vi "calculate_white-bias_jsc.vi"(9 "wavelengths":dbl[](array[numeric]), 10 "eqe measurements":dbl[](array[numeric]), 11 "am1.5 jsc (mA/cm^2)":dbl) -> (2 "white bias (# of suns)":dbl)   [LabVIEW 2018]
uses:
  <vilib>/Analysis/2dsp.llb/Integral Method.ctl
  <vilib>/Analysis/8numeric.llb/1D Numeric Integration.vi
  <vilib>/Utility/file.llb/Read Delimited Spreadsheet (DBL).vi
  <vilib>/gmath/NI_Gmath.lvlib
  <vilib>/Analysis/NI_AALPro.lvlib
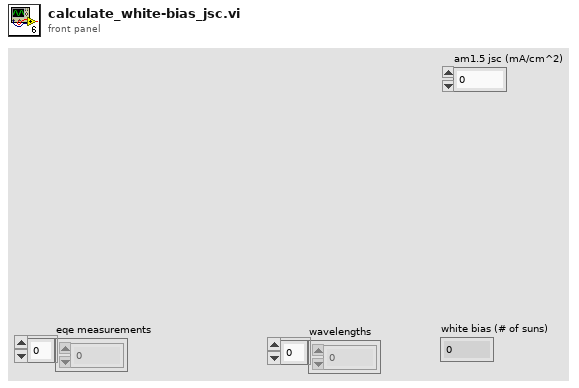
[diagram p1: front panel]
types:
  T1 = typedef "NI_AALPro.lvlib/Integral Method.ctl" = i32
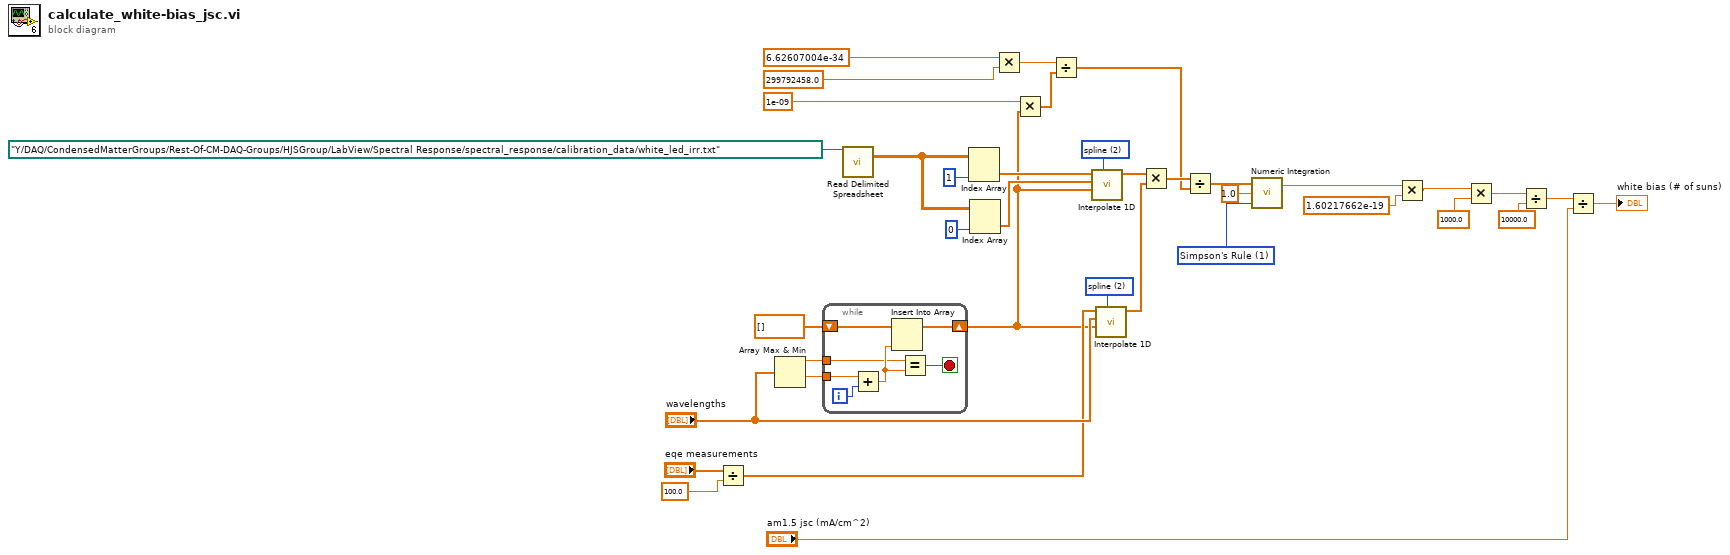
[diagram p0: block diagram]
diagram:
  w10 = 2 items=["nearest", "linear", "spline", "cubic Hermite", "Lagrange"] ("method")
  w18 = T1 1 items=["Trapezoidal Rule", "Simpson's Rule", "Simpson's 3/8 Rule", "Bode Rule"] ("integration method")
  w31 = 2 items=["nearest", "linear", "spline", "cubic Hermite", "Lagrange"] ("method")
  n1 = Divide(x="eqe measurements", y=100.0) -> (x/y=w7:dbl[])
  n2 = Array Max & Min(array="wavelengths") -> (max value=w11:dbl, min value=w13:dbl)  [unwired: 2 out]
  n3 = while {
    tunnel: w13 -> [w43]
    shift-right: [w41] -> w6
    shift-left: dbl[] [] ("wavelengths") -> [w42]
    tunnel: w11 -> [w38]
    i -> [w44]
    stop <- w40 stop-if-true
    n4 = Add(x=w43, y=w44) -> (x+y=w39:dbl)
    n5 = Insert Into Array(array=w42, new element=w39) -> (w41:dbl[])  [unwired: 1 in]
    n6 = Equal?(x=w38, y=w39) -> (x = y?=w40:bool)
  }
  n7 = call-poly <vilib>:"Read Delimited Spreadsheet.vi"("file path (dialog if empty)"=path "Y:/DAQ/CondensedMatterGroups/Rest-Of-CM-DAQ-Groups/HJSGroup/LabView/Spectral Response/spectral_response/calibration_data/white_led_irr.txt" ("AM1.5G file path")) -> ("all rows"=w35:dbl[][])  [unwired: 9 in, 5 out]
  n8 = Index Array(array=w35, index (col)=1 ("disabled index (col)")) -> (element=w33:dbl[])  [unwired: 1 in]
  n9 = Index Array(array=w35, index (col)=0 ("index")) -> (element=w32:dbl[])  [unwired: 1 in]
  n10 = Multiply(x=6.62607004e-34, y=299792458.0) -> (x*y=w28:dbl)
  n11 = Multiply(x=1e-09 ("y"), y=w6) -> (x*y=w27:dbl[])
  n12 = Divide(x=w28, y=w27) -> (x/y=w21:dbl[])
  n13 = call <vilib>:"Interpolate 1D.vi"("method"=w31, "xi"=w6, "X"=w32, "Y"=w33) -> ("yi"=w25:dbl[])  [unwired: 5 in, 2 out]
  n14 = call <vilib>:"Interpolate 1D.vi"("method"=w10, "xi"=w6, "X"="wavelengths", "Y"=w7) -> ("yi"=w9:dbl[])  [unwired: 5 in, 2 out]
  n15 = Multiply(x=w25, y=w9) -> (x*y=w22:dbl[])
  n16 = Divide(x=w22, y=w21) -> (x/y=w19:dbl[])
  n17 = call-poly <vilib>:"Numeric Integration.vi"("integration method"=w18, "dt"=1.0, "Input Array"=w19) -> ("result"=w20:dbl)  [unwired: 1 out]
  n18 = Multiply(x=w20, y=1.60217662e-19) -> (x*y=w2:dbl)
  n19 = Multiply(x=w2, y=1000.0) -> (x*y=w4:dbl)
  n20 = Divide(x=w4, y=10000.0) -> (x/y=w1:dbl)
  n21 = Divide(x=w1, y="am1.5 jsc (mA/cm^2)") -> (x/y=→"white bias (# of suns)":dbl)
